vi "REACTOR__SET_ALICATS.vi"(6 "error in (no error)":errorcluster, 7 "SERIAL Alicats":T1) -> (0 "error out":errorcluster, 1 "%MFCf":dbl[](array[numeric]) format="%.1g", 3 "Cancelled?":bool)   [LabVIEW 2017]
doc: "Use this template to create a dialog box. This template polls the state of the buttons on the front panel and does not use events. Use the Dialog Using Events template (not available in Base package) to create a dialog box with event handling."
uses:
  SERIAL ALICATS/__s_TablaAlicats.ctl
panel:
  in  "SP4 2":dbl format="%.2f"
  in  "SP3 2":dbl format="%.2f"
  in  "SP2 2":dbl format="%.2f"
  in  "SP1 2":dbl format="%.2f"
  in  "Cancel":bool
  in  "OK":bool
  # "FLUJOS DE GAS"
  # "NUEVO"
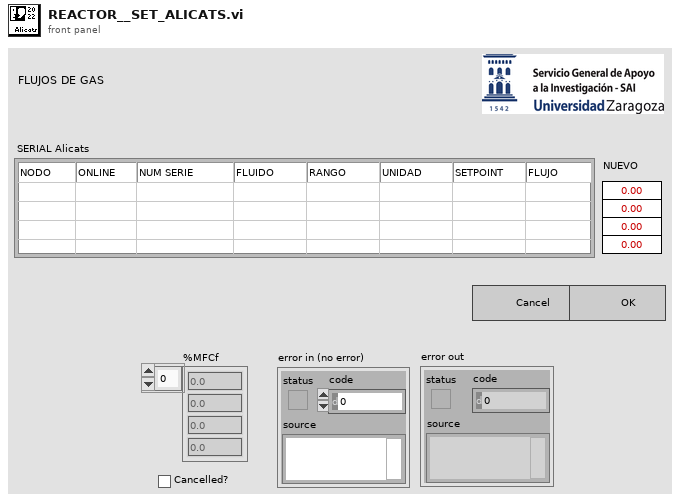
[diagram p1: front panel]
types:
  T1 = typedef "__s_TablaAlicats.ctl" = string[][]
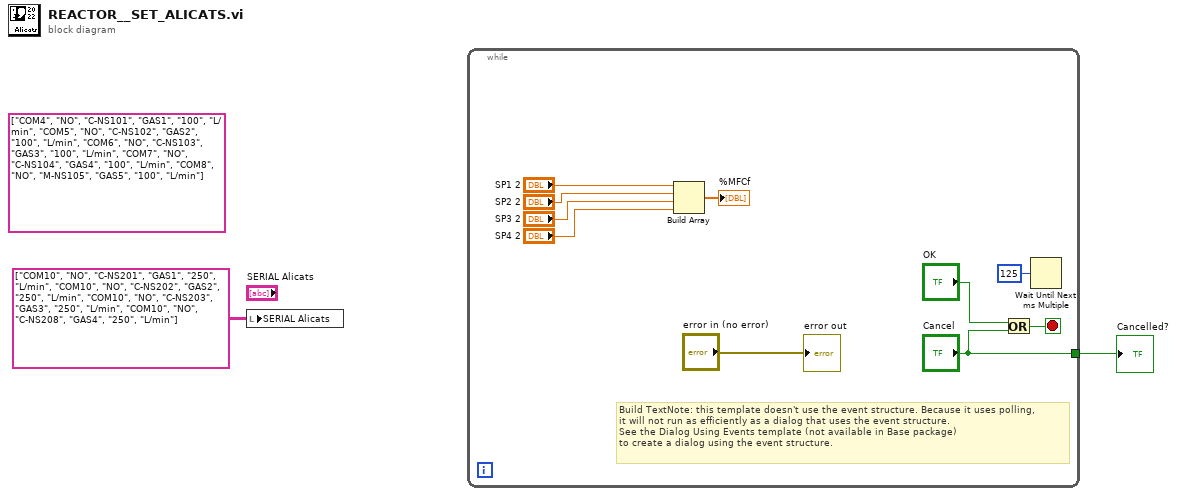
[diagram p0: block diagram]
diagram:
  (unwired) T1 [["COM4", "NO", "C-NS101", "GAS1", "100", "L/min"], ["COM5", "NO", "C-NS102", "GAS2", "100", "L/min"], ["COM6", "NO", "C-NS103", "GAS3", "100", "L/min"], ["COM7", "NO", "C-NS104", "GAS4", "100", "L/min"], ["COM8", "NO", "M-NS105", "GAS5", "100", "L/min"]] ("SERIAL Alicats")
  n1 = local write "SERIAL Alicats"(T1 [["COM10", "NO", "C-NS201", "GAS1", "250", "L/min"], ["COM10", "NO", "C-NS202", "GAS2", "250", "L/min"], ["COM10", "NO", "C-NS203", "GAS3", "250", "L/min"], ["COM10", "NO", "C-NS208", "GAS4", "250", "L/min"]] ("SERIAL Alicats")) -> ()
  n2 = while {
    tunnel: ["Cancel"] -> w2
    stop <- w11 stop-if-true
    # "Build TextNote: this template doesn't use the event structure. Because it uses polling, \nit will not run as efficiently as a dialog that uses the event structure.\nSee the Dialog Using Events template (not available in Base package) \nto create a dialog using the event structure."
    n3 = Build Array("SP1 2", "SP2 2", "SP3 2", "SP4 2") -> (→"%MFCf":dbl[])
    n4 = Or(x="OK", y="Cancel") -> (x .or. y?=w11:bool)
    n5 = Wait Until Next ms Multiple(millisecond multiple=u32 125) -> ()  [unwired: 1 out]
    "error out" <- "error in (no error)"
  }
  "Cancelled?" <- w2
